vi "Check1.vi"() -> ()   [LabVIEW 2019]
panel:
  in  "setpoint 2":cluster{dbl, dbl, dbl}(slide)={350.0, 0.0, 0.0} caption="oC" scale=0.0..500.0 scale format="%#.1f"
  in  "SP":dbl
  in  "SP Set":dbl
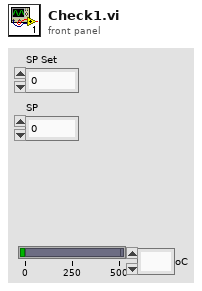
[diagram p1: front panel]
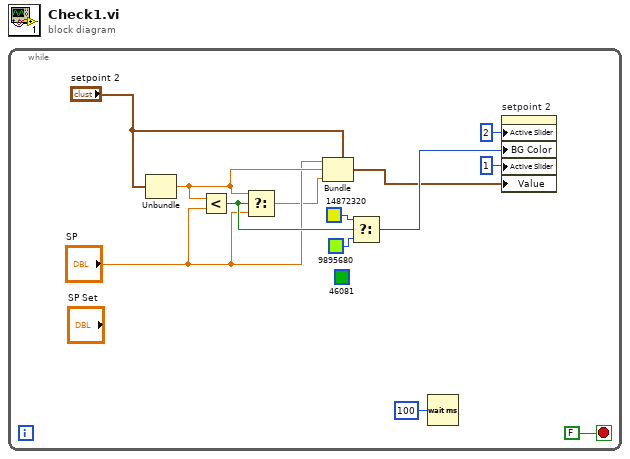
[diagram p0: block diagram]
diagram:
  n1 = while {
    stop <- FALSE stop-if-true
    (unwired) u32 46081
    n2 = Unbundle("setpoint 2") -> (w6:dbl)  [unwired: 2 out]
    n3 = Less?(x=w6, y="SP") -> (x < y?=w13:bool)
    n4 = Select(t=w6, s=w13, f="SP") -> (s? t:f=w4:dbl)
    n5 = Bundle(cluster="setpoint 2", "SP", w6, w4) -> (w7:cluster{dbl, dbl, dbl})
    n6 = Select(t=u32 14872320, s=w13, f=u32 9895680) -> (s? t:f=w9:u32)
    n7 = Wait (ms)(milliseconds to wait=u32 100) -> ()  [unwired: 1 out]
    n8 = property on="setpoint 2" class="Slide (strict)"("Active Slider"=2, "BG Color"=w9, "Active Slider"=1, "Value"=w7) -> ()  [unwired: 2 in, 2 out]
  }
